vi "errorHandler.vi"(7 "show popup":bool, 9 "language":i32, 10 "error number":i8, 11 "connection ID":refnum<k5>) -> (0 "error out":errorcluster, 3 "connection ID":refnum<k5>)   [LabVIEW 2015]
panel:
  in  "Set Command":string="com.attocube.system.errorNumberToString"
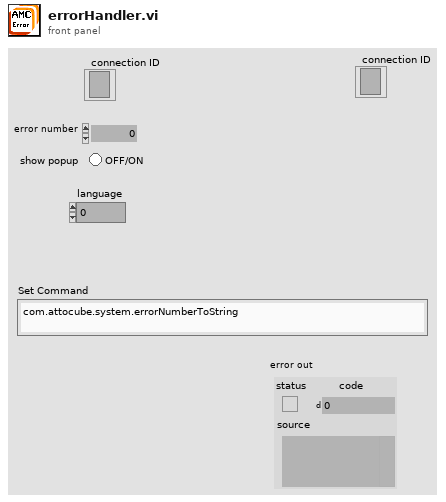
[diagram p1: front panel]
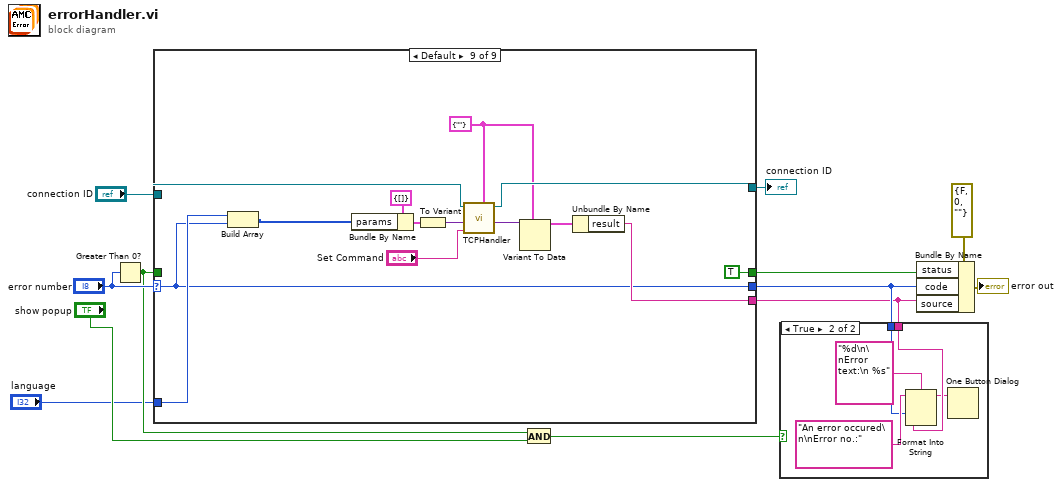
[diagram p0: block diagram]
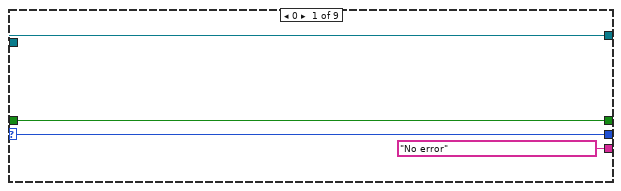
[diagram p3: hidden frame]
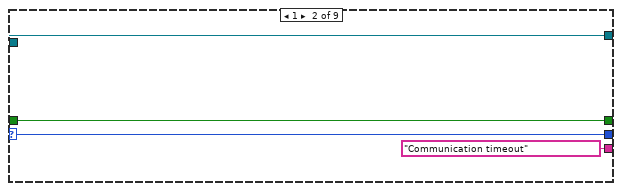
[diagram p4: hidden frame]
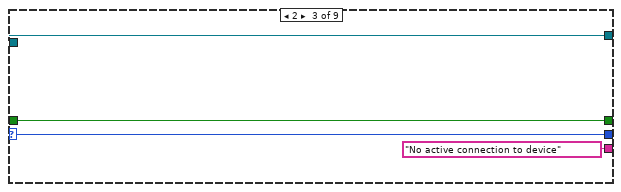
[diagram p5: hidden frame]
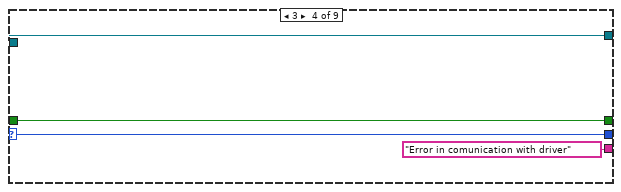
[diagram p6: hidden frame]
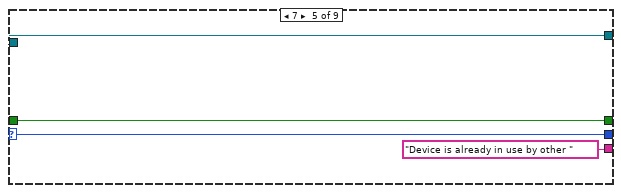
[diagram p7: hidden frame]
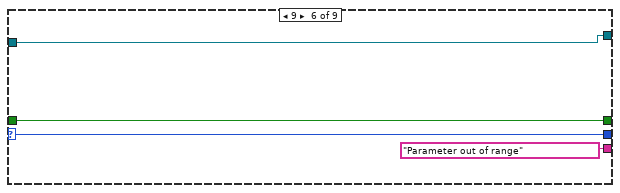
[diagram p8: hidden frame]
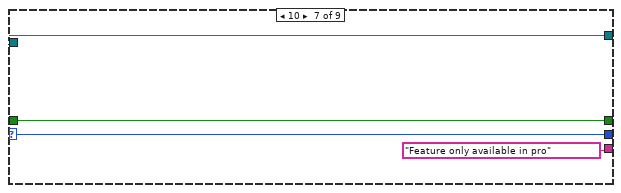
[diagram p9: hidden frame]
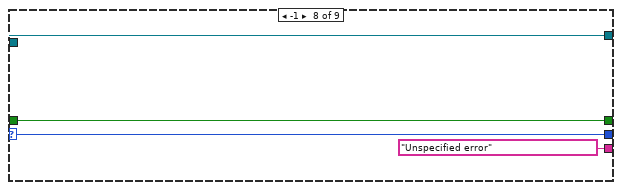
[diagram p10: hidden frame]
diagram:
  n1 = Greater Than 0?(x="error number") -> (x > 0?=w8:bool)
  n2 = case shown="Default" "error number" {
    selector: "error number" -> [w15 w20 w23 w27 w31 w35 w39 w43 w45]
    tunnel: ["No error" "Communication timeout" "No active connection to device" "Error in comunication with driver" "Device is already in use by other " "Parameter out of range" "Feature only available in pro" "Unspecified error" w48] -> w9
    tunnel: [w15 w20 w23 w27 w31 w35 w39 w43 w45] -> w10
    tunnel: [w14 w19 w22 w28 w32 w36 w38 w44 TRUE] -> w11
    tunnel: w8 -> [w14 w19 w22 w28 w32 w36 w38 w44 _]
    tunnel: "language" -> [_ _ _ _ _ _ _ _ w46]
    tunnel: "connection ID" -> [w13 w17 w21 w25 w29 w33 w37 w41 w57]
    tunnel: [w13 w17 w21 w25 w29 w33 w37 w41 w56] -> w4
    frame 0 {
    }
    frame 1 {
    }
    frame 2 {
    }
    frame 3 {
    }
    frame 7 {
    }
    frame 9 {
    }
    frame 10 {
    }
    frame -1 {
    }
    frame Default {
      w47 = cluster{"result":string} {"result"=""} ("input cluster")
      n3 = Build Array(w46, w45) -> (w52:i32[])
      n4 = Bundle By Name(cluster=cluster{"params":i64[]} {"params"=[]} ("input cluster"), "params"=w52) -> (w54:cluster{"params":i64[]})
      n5 = To Variant(anything=w54) -> (Variant=w53:variant)
      n6 = call "TCPHandler.vi"("result Types"=w47, "method"="Set Command", "params"=w53, "connection ID"=w57) -> ("result"=w49:variant, "connection ID"=w56:refnum<k5>)  [unwired: 5 in, 1 out]
      n7 = Variant To Data(type=w47, Variant=w49) -> (data=w50:cluster{"result":string})  [unwired: 1 in, 1 out]
      n8 = Unbundle By Name(w50) -> ("result"=w48:string)
    }
  }
  "connection ID" <- w4
  n9 = And(x=w8, y="show popup") -> (x .and. y?=w6:bool)
  n10 = case shown="True" w6 {
    tunnel: w10 -> [_ w62]
    tunnel: w9 -> [_ w60]
    frame False {
    }
    frame True {
      n11 = Format Into String(format string="%d\n\nError text:\n %s", initial string="An error occured\n\nError no.:", w62, w60) -> (resulting string=w59:string)  [unwired: 1 in, 1 out]
      n12 = One Button Dialog(message=w59) -> ()  [unwired: 1 in, 1 out]
    }
  }
  n13 = Bundle By Name(cluster=errorcluster {"status"=FALSE, "code"=0, "source"=""} ("error in"), "status"=w11, "code"=w10, "source"=w9) -> (→"error out":errorcluster)
